vi "Main.vi"(10 "Caller Return Queue":refnum<queue>, 11 "Connection Handler in":refnum<class "Connection Handler.lvclass">) -> ()   [LabVIEW 2017, in "Network Interface.lvlib" / "Connection Handler.lvclass"]
uses:
  <vilib>/gpm_packages/@cs/Network-sink/Source/Network Interface/Connection Handler/Connection Handler.lvclass
  <vilib>/gpm_packages/@cs/Network-sink/Source/Network Interface/Message Queue/Message Queue.lvclass
  <vilib>/gpm_packages/@cs/Network-sink/Source/Network Interface/Connection Handler/Connection Handler.lvclass/Connection Handler.ctl
  <vilib>/gpm_packages/@cs/Network-sink/Source/Network Interface/Connection Handler/Message Names ENUM.ctl
  <vilib>/gpm_packages/@cs/Network-sink/Source/Network Interface/Message Queue/Message Queue.lvclass/Message Queue.ctl
  <vilib>/gpm_packages/@cs/Network-sink/Source/Network Interface/Connection Handler/Synchronous Write Request.ctl
  e36f3f40-7fc8-477c-977b-0dc36704a1f5.vi
  65cd8ff4-e8dd-4385-b791-2b2ca0a6875d.vi
  <vilib>/gpm_packages/@cs/Network-sink/Source/Network Interface/Message Queue/Protected Enqueue.vi
  <vilib>/gpm_packages/@cs/Network-sink/Source/Network Interface/Message Queue/Dequeue Message.vi
  <vilib>/gpm_packages/@cs/Network-sink/Source/Network Interface/IConnection/IConnection.lvclass
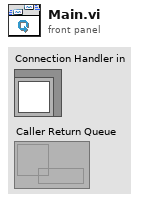
[diagram p1: front panel]
types:
  T1 = typedef "Network Interface.lvlib/Connection Handler.lvclass/Synchronous Write Request.ctl" = cluster{"Data To Write":string, "Return Queue":refnum<queue>}
  T2 = typedef "Network Interface.lvlib/Connection Handler.lvclass/Message Names ENUM.ctl" = enum16{"Transmit Message", "Stop"}
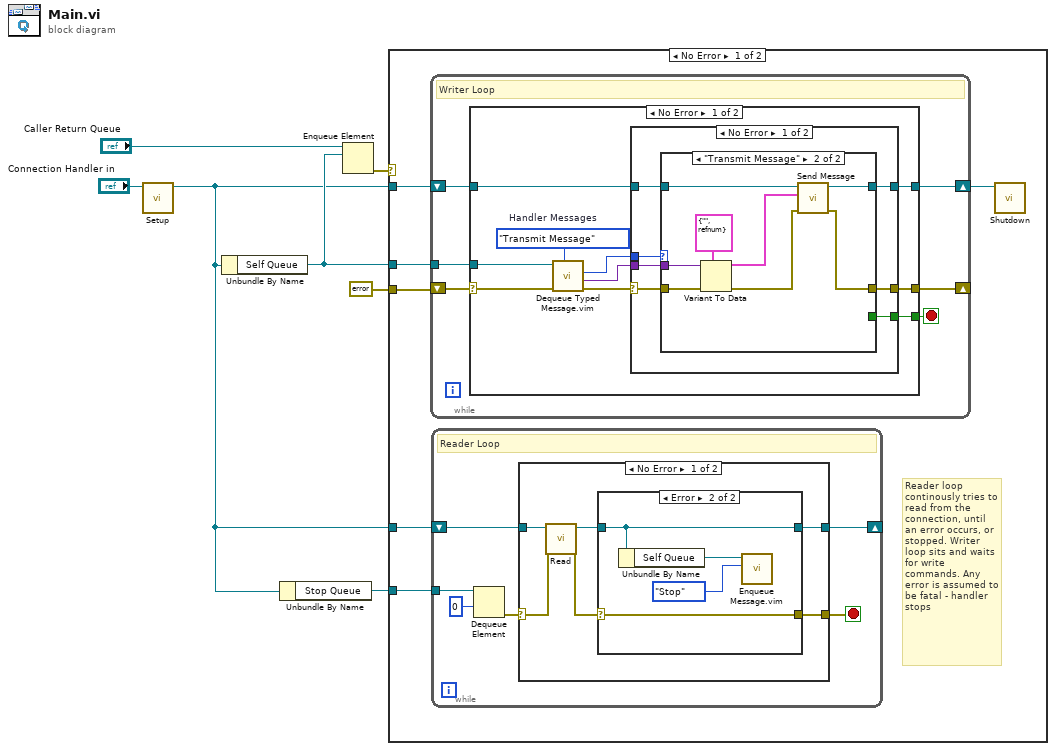
[diagram p0: block diagram]
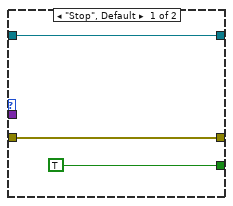
[diagram p2: hidden frame]
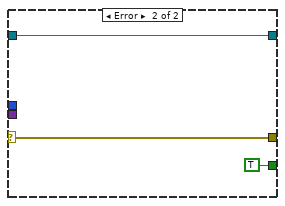
[diagram p3: hidden frame]
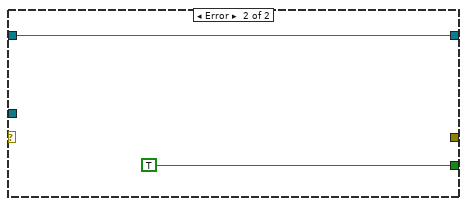
[diagram p4: hidden frame]
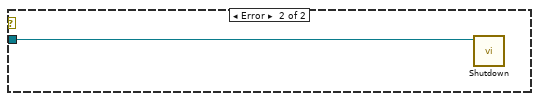
[diagram p7: hidden frame]
diagram:
  n1 = call <vilib>:"Setup.vi"("Connection Handler in"="Connection Handler in") -> ("Connection Handler out"=w2:refnum<class "Connection Handler.lvclass">)  [unwired: 10 in]
  n2 = Unbundle By Name(w2) -> ("Self Queue"=w4:refnum<class "Message Queue.lvclass">)
  n3 = Unbundle By Name(w2) -> ("Stop Queue"=w6:refnum<queue>)
  n4 = Enqueue Element(queue="Caller Return Queue", element=w4) -> (error out=w3:errorcluster)  [unwired: 2 in, 2 out]
  n5 = case shown="No Error" w3 {
    tunnel: w2 -> [w13 w73]
    tunnel: w6 -> [w12 _]
    tunnel: w4 -> [w11 _]
    tunnel: w2 -> [w10 _]
    tunnel: errorcluster {"status"=FALSE, "code"=0, "source"=""} ("error out") -> [w9 _]
    frame No Error {
      # "Reader loop continously tries to read from the connection, until an error occurs, or stopped. Writer loop sits and waits for write commands. Any error is assumed to be fatal - handler stops"
      n6 = while {
        shift-right: [w16] -> w8
        shift-left: w13 -> [w17]
        shift-right: [w19] -> _
        shift-left: w9 -> [w18]
        tunnel: w11 -> [w14]
        stop <- w15 stop-if-true
        # "Writer Loop"
        n7 = case shown="No Error" w18 {
          selector: w18 -> [w25 _]
          tunnel: [w29 _] -> w19
          tunnel: w17 -> [w28 w52]
          tunnel: [w27 w52] -> w16
          tunnel: [w26 TRUE] -> w15
          tunnel: w14 -> [w24 _]
          frame No Error {
            w21 = Message_Names_ENUM."Transmit Message"  # Handler Messages
            n8 = call "Dequeue Typed Message.vim"("Type"=w21, "error in (no error)"=w25, "Message Queue in"=w24) -> ("error out"=w23:errorcluster, "Data"=w22:variant, "Msg"=w20:T2)  [unwired: 4 in, 2 out]
            n9 = case shown="No Error" w23 {
              selector: w23 -> [w32 w50]
              tunnel: [w36 w50] -> w29
              tunnel: w28 -> [w35 w49]
              tunnel: [w34 w49] -> w27
              tunnel: [w33 TRUE] -> w26
              tunnel: w22 -> [w31 _]
              tunnel: w20 -> [w30 _]
              frame No Error {
                n10 = case shown="\"Transmit Message\"" w30 {
                  tunnel: [w37 w45] -> w36
                  tunnel: w35 -> [w39 w47]
                  tunnel: [w39 w46] -> w34
                  tunnel: [TRUE _] -> w33
                  tunnel: w31 -> [_ w41]
                  tunnel: w32 -> [w37 w40]
                  frame "Stop", Default {
                  }
                  frame "Transmit Message" {
                    n11 = Variant To Data(error in=w40, type=T1 {"Data To Write"="", "Return Queue"=refnum} ("Write Request"), Variant=w41) -> (data=w42:T1, error out=w44:errorcluster)
                    n12 = call <vilib>:"Send Message.vi"("error in (no error)"=w44, "Write Request"=w42, "Connection Handler in"=w47) -> ("error out"=w45:errorcluster, "Connection Handler out"=w46:refnum<class "Connection Handler.lvclass">)  [unwired: 7 in]
                  }
                }
              }
              frame Error {
              }
            }
          }
          frame Error {
          }
        }
      }
      n13 = while {
        shift-right: [w57] -> _
        shift-left: w10 -> [w58]
        tunnel: w12 -> [w55]
        stop <- w56 stop-if-true
        # "Reader Loop"
        n14 = Dequeue Element(queue=w55, timeout in ms (-1)=0) -> (error out=w53:errorcluster)  [unwired: 1 in, 3 out]
        n15 = case shown="No Error" w53 {
          selector: w53 -> [w59 w71]
          tunnel: w58 -> [w64 w72]
          tunnel: [w61 w72] -> w57
          tunnel: [w60 w71] -> w56
          frame No Error {
            n16 = call <vilib>:"Read.vi"("error in (no error)"=w59, "Connection Handler in"=w64) -> ("error out"=w63:errorcluster, "Connection Handler out"=w62:refnum<class "Connection Handler.lvclass">)  [unwired: 8 in]
            n17 = case shown="Error" w63 {
              selector: w63 -> [w65 w68]
              tunnel: [w66 w69] -> w61
              tunnel: w62 -> [w66 w69]
              tunnel: [w65 w68] -> w60
              frame No Error {
              }
              frame Error {
                n18 = Unbundle By Name(w69) -> ("Self Queue"=w70:refnum<class "Message Queue.lvclass">)
                n19 = call "Enqueue Message.vim"("Msg"=Message_Names_ENUM."Stop", "Message Queue in"=w70) -> ()  [unwired: 8 in, 2 out]
              }
            }
          }
          frame Error {
          }
        }
      }
      n20 = call <vilib>:"Shutdown.vi"("Connection Handler in"=w8) -> ()  [unwired: 11 in]
    }
    frame Error {
      n21 = call <vilib>:"Shutdown.vi"("Connection Handler in"=w73) -> ()  [unwired: 11 in]
    }
  }
